vi "BrainStemExample_PortToggle.vi"() -> ()   [LabVIEW 2015, in "BrainStem4LabView.lvlib"]
uses:
  BrainStem_DLL_Import/BrainStem4LabView.lvlib
panel:
  out "Port 0 Voltage":u32
  out "Port 3 Current":u32
  out "Port 2 Current":u32
  out "Port 1 Current":u32
  out "Port 0 Current":u32
  out "Port 3 Voltage":u32
  out "Port 2 Voltage":u32
  out "Port 1 Voltage":u32
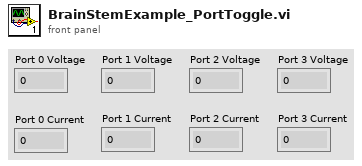
[diagram p1: front panel]
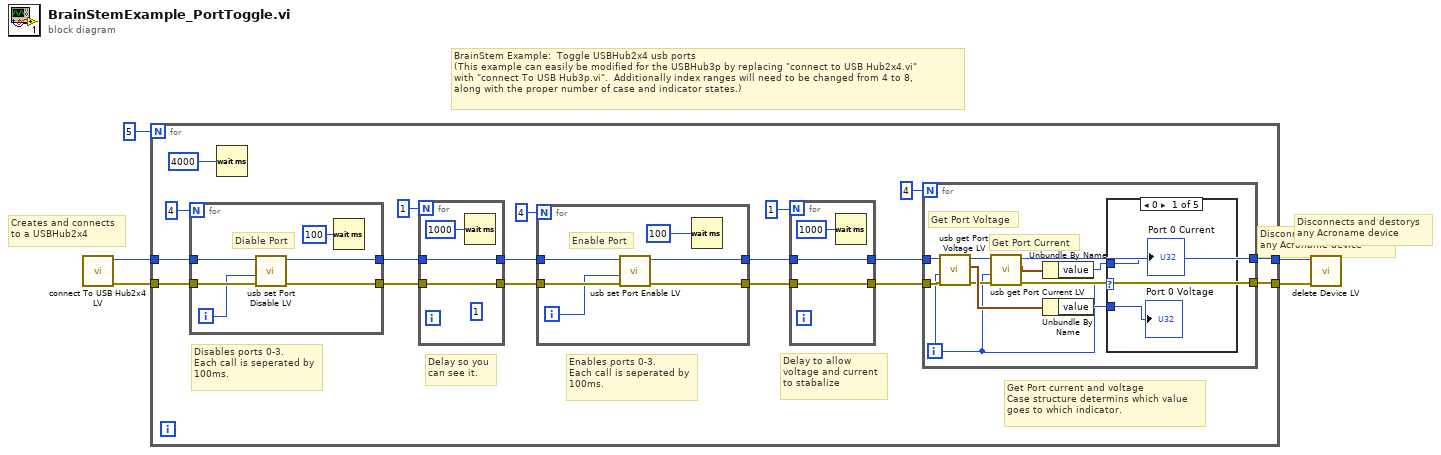
[diagram p0: block diagram]
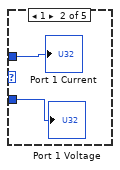
[diagram p2: hidden frame]
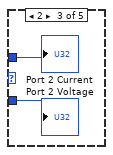
[diagram p3: hidden frame]
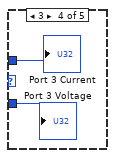
[diagram p4: hidden frame]
diagram:
  # "Disconnects and destorys\nany Acroname device"
  # "Disconnects and destorys\nany Acroname device"
  # "Creates and connects\nto a USBHub2x4"
  # "BrainStem Example:  Toggle USBHub2x4 usb ports\n(This example can easily be modified for the USBHub3p by replacing \"connect to USB Hub2x4.vi\"\nwith \"connect To USB Hub3p.vi\".  Additionally index ranges will need to be changed from 4 to 8, \nalong with the proper number of case and indicator states.)"
  n1 = call "connect To USB Hub2x4 LV.vi"() -> ("error out"=w3:errorcluster, "id out"=w5:i32)  [unwired: 9 in, 1 out]
  n2 = for {
    N: 5 -> [_]
    tunnel: w5 -> [w21]
    tunnel: [w12] -> w4
    tunnel: w3 -> [w20]
    tunnel: [w11] -> w2
    (unwired) 1
    # "Get Port current and voltage\nCase structure determins which value\ngoes to which indicator."
    # "Delay to allow\nvoltage and current\nto stabalize"
    # "Enables ports 0-3.\nEach call is seperated by\n100ms."
    # "Disables ports 0-3.\nEach call is seperated by\n100ms."
    # "Delay so you\ncan see it."
    n3 = for {
      N: 4 -> [_]
      tunnel: w21 -> [w60]
      tunnel: [w59] -> w16
      tunnel: w20 -> [w58]
      tunnel: [w57] -> w18
      i -> [w55]
      # "Diable Port"
      n4 = call "usb set Port Disable LV.vi"("error in (no error)"=w58, "port"=w55, "id"=w60) -> ("error out"=w57:errorcluster, "id out"=w59:i32)  [unwired: 6 in, 1 out]
      n5 = Wait (ms)(milliseconds to wait=100) -> ()  [unwired: 1 out]
    }
    n6 = Wait (ms)(milliseconds to wait=4000) -> ()  [unwired: 1 out]
    n7 = for {
      N: 1 -> [_]
      tunnel: [w48] -> w19
      tunnel: w18 -> [w48]
      tunnel: [w47] -> w17
      tunnel: w16 -> [w47]
      n8 = Wait (ms)(milliseconds to wait=1000) -> ()  [unwired: 1 out]
    }
    n9 = for {
      N: 4 -> [_]
      tunnel: w17 -> [w54]
      tunnel: [w53] -> w10
      tunnel: w19 -> [w52]
      tunnel: [w51] -> w9
      i -> [w49]
      # "Enable Port"
      n10 = call "usb set Port Enable LV.vi"("error in (no error)"=w52, "port"=w49, "id"=w54) -> ("error out"=w51:errorcluster, "id out"=w53:i32)  [unwired: 6 in, 1 out]
      n11 = Wait (ms)(milliseconds to wait=100) -> ()  [unwired: 1 out]
    }
    n12 = for {
      N: 1 -> [_]
      tunnel: [w26] -> w7
      tunnel: w9 -> [w26]
      tunnel: [w25] -> w8
      tunnel: w10 -> [w25]
      n13 = Wait (ms)(milliseconds to wait=1000) -> ()  [unwired: 1 out]
    }
    n14 = for {
      N: 4 -> [_]
      tunnel: w8 -> [w31]
      tunnel: w7 -> [w30]
      tunnel: [w29] -> w12
      tunnel: [w28] -> w11
      i -> [w27]
      # "Get Port Current"
      # "Get Port Voltage"
      n15 = call "usb get Port Voltage LV.vi"("error in (no error)"=w30, "port"=w27, "id"=w31) -> ("error out"=w35:errorcluster, "result out"=w36:cluster{"value":i32, "error":i32}, "id out"=w34:i32)  [unwired: 6 in]
      n16 = call "usb get Port Current LV.vi"("error in (no error)"=w35, "port"=w27, "id"=w34) -> ("error out"=w28:errorcluster, "result out"=w37:cluster{"value":i32, "error":i32}, "id out"=w29:i32)  [unwired: 6 in]
      n17 = Unbundle By Name(w37) -> ("value"=w32:i32)
      n18 = Unbundle By Name(w36) -> ("value"=w33:i32)
      n19 = case shown="0" w27 {
        tunnel: w33 -> [w39 w40 w42 w45 _]
        tunnel: w32 -> [w38 w41 w43 w44 _]
        frame 0 {
          "Port 0 Current" <- w38
          "Port 0 Voltage" <- w39
        }
        frame 1 {
          "Port 1 Voltage" <- w40
          "Port 1 Current" <- w41
        }
        frame 2 {
          "Port 2 Voltage" <- w42
          "Port 2 Current" <- w43
        }
        frame 3 {
          "Port 3 Current" <- w44
          "Port 3 Voltage" <- w45
        }
        frame 4, Default {
        }
      }
    }
  }
  n20 = call "delete Device LV.vi"("error in (no error)"=w2, "id"=w4) -> ()  [unwired: 8 in, 2 out]
